vi "CAL-Get Max SPL (tone, 1D).vi"(0 "Speaker name":path, 7 "Frequency (kHz)":dbl[](array[numeric]), 11 "error in (no error)":errorcluster) -> (8 "Max SPL":dbl[](array[numeric]), 15 "error out":errorcluster)   [LabVIEW 2020]
uses:
  PXI DAQ VIs/DAQ Engine VIs/PXI Globals.vi
  Utility VIs/Math VIs/Linear to dB (scalar).vi
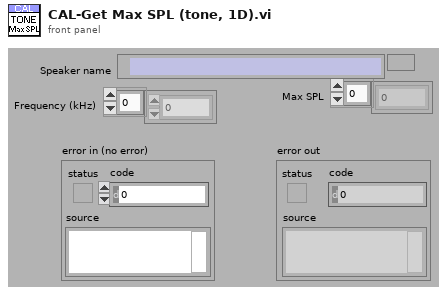
[diagram p1: front panel]
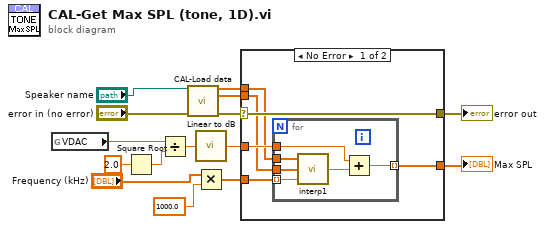
[diagram p0: block diagram]
diagram:
  n1 = global read "PXI Globals.vi" "VDAC"() -> (w3:dbl)
  n2 = Square Root(x=2.0 ("y")) -> (sqrt(x)=w7:dbl)
  n3 = Divide(x=w3, y=w7) -> (x/y=w9:dbl)
  n4 = call "CAL-Load data.vi"("user path"="Speaker name", "error in (no error)"="error in (no error)") -> ("Frequency (Hz)"=w12:dbl[], "Mag"=w1:dbl[], "error out"=w14:errorcluster)  [unwired: 6 in, 5 out]
  n5 = call-poly "Linear to dB.vi"("Linear"=w9) -> ("dB"=w10:dbl)
  n6 = Multiply(x="Frequency (kHz)", y=1000.0 ("x")) -> (x*y=w6:dbl[])
  n7 = case shown="No Error" w14 {
    selector: w14 -> [w21 w28]
    tunnel: [w21 w28] -> w13
    tunnel: w12 -> [w17 _]
    tunnel: w6 -> [w20 _]
    tunnel: [w19 _] -> w11
    tunnel: w10 -> [w18 _]
    tunnel: w1 -> [w16 _]
    frame No Error {
      n8 = for {
        tunnel: w20 -> [w27] mode=indexing
        tunnel: [w25] -> w19 mode=indexing
        tunnel: w18 -> [w24]
        tunnel: w17 -> [w23]
        tunnel: w16 -> [w22]
        n9 = call "interp1.vi"("X"=w23, "Y"=w22, "U"=w27) -> ("V"=w26:dbl)  [unwired: 2 in]
        n10 = Add(x=w24, y=w26) -> (x+y=w25:dbl)
      }
    }
    frame Error {
    }
  }
  "error out" <- w13
  "Max SPL" <- w11
